vi "Get_Response_Type.vi"(8 "error in (no error)":errorcluster, 11 "Asana in":refnum<class "Asana.lvclass">) -> (0 "error out":errorcluster, 3 "Asana out":refnum<class "Asana.lvclass">)   [LabVIEW 2016, in "Asana.lvclass"]
uses:
  Asana.lvclass
  Asana.lvclass/Asana.ctl
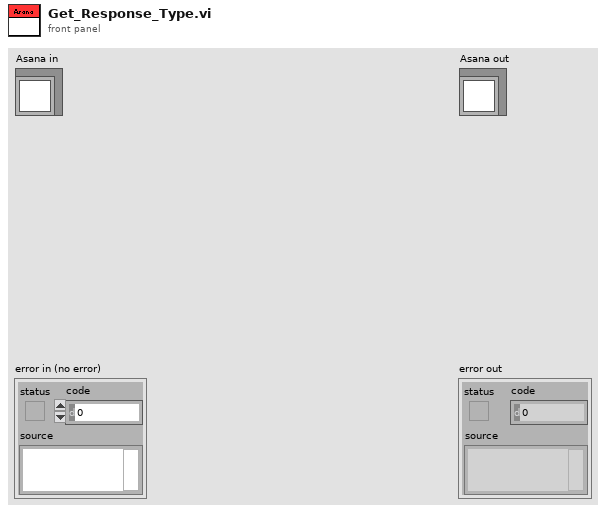
[diagram p1: front panel]
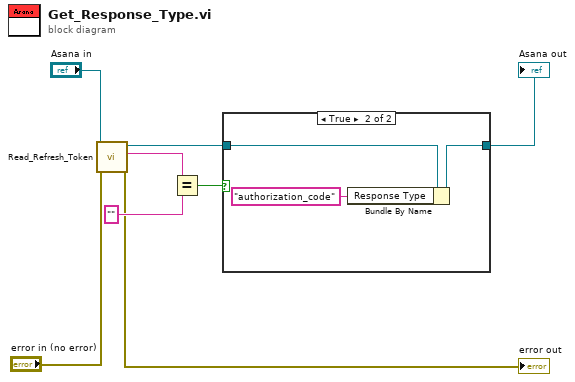
[diagram p0: block diagram]
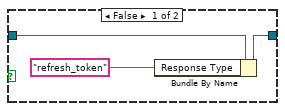
[diagram p2: hidden frame]
diagram:
  n1 = call-dynamic "Read_Refresh_Token.vi"("error in (no error)"="error in (no error)", "Asana in"="Asana in") -> ("error out"=→"error out":errorcluster, "Refresh Token"=w4:string, "Asana out"=w7:refnum<class "Asana.lvclass">)  [unwired: 7 in]
  n2 = Equal?(x=w4, y="") -> (x = y?=w5:bool)
  n3 = case shown="True" w5 {
    tunnel: w7 -> [w11 w14]
    tunnel: [w10 w13] -> w2
    frame False {
      n4 = Bundle By Name(cluster=w11, "Response Type"="refresh_token") -> (w10:refnum<class "Asana.lvclass">)
    }
    frame True {
      n5 = Bundle By Name(cluster=w14, "Response Type"="authorization_code") -> (w13:refnum<class "Asana.lvclass">)
    }
  }
  "Asana out" <- w2
